vi "READ DUBAS DATA.vi"(7 "STATES":T1=enum."CLOSE", 8 "error in (no error)":errorcluster) -> (0 "error out":errorcluster, 3 "BUBAS DATA":dbl[](array[numeric]) caption="data" format="%.2f")   [LabVIEW 2018]
uses:
  Controls/DUBAS FGV STATES.ctl
  <vilib>/xnet/xnet.llb/XNET Create Session (Signal Input Single-point).vi
  <vilib>/xnet/xnet.llb/XNET Read (Signal Single-point).vi
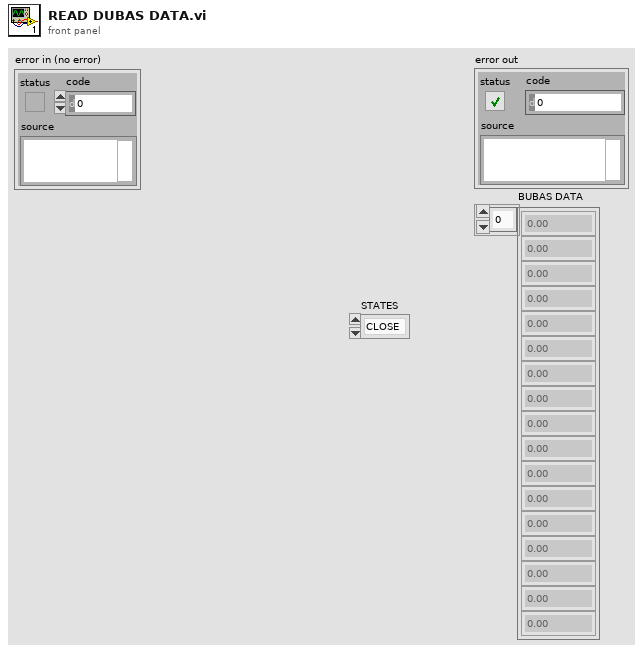
[diagram p1: front panel]
types:
  T1 = typedef "DUBAS FGV STATES.ctl" = enum16{"OPEN REF", "READ DATA", "CLOSE"}
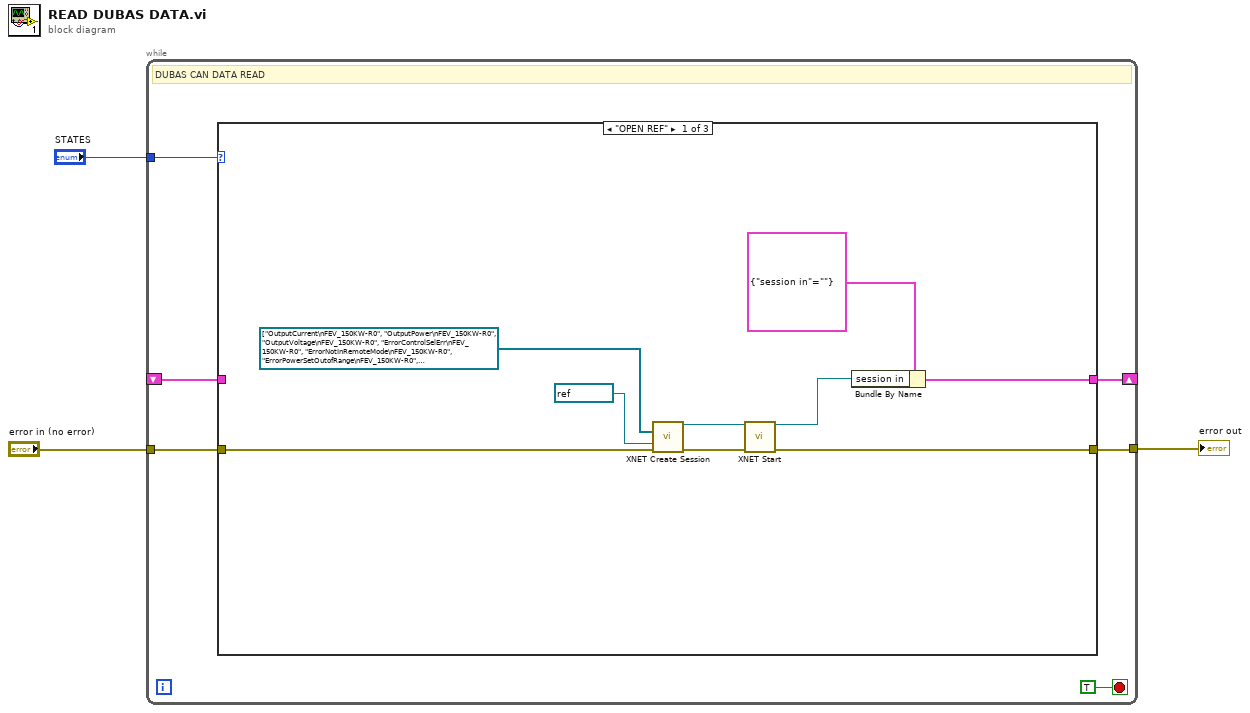
[diagram p0: block diagram]
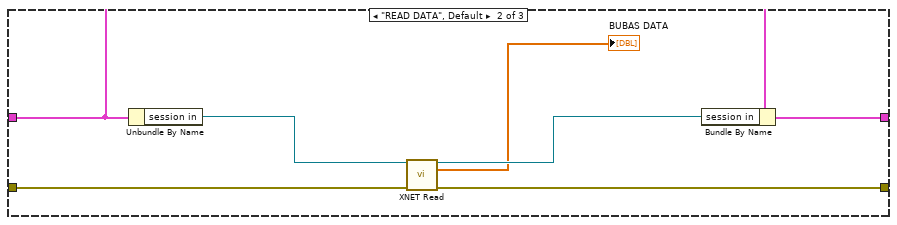
[diagram p2: hidden frame]
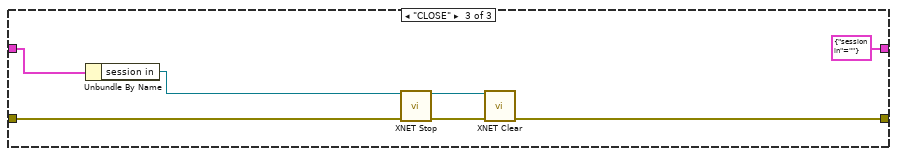
[diagram p3: hidden frame]
diagram:
  n1 = while {
    tunnel: "STATES" -> [w8]
    tunnel: "error in (no error)" -> [w7]
    tunnel: [w6] -> w1
    shift-right: [w5] -> _
    shift-left: _ -> [w4]
    stop <- TRUE stop-if-true
    # "DUBAS CAN DATA READ"
    n2 = case shown="\"OPEN REF\"" w8 {
      tunnel: w7 -> [w14 w25 w32]
      tunnel: [w13 w24 w27] -> w6
      tunnel: [w10 w20 cluster{"session in":refnum<k21>} {"session in"=""}] -> w5
      tunnel: w4 -> [_ w22 w31]
      frame "OPEN REF" {
        n3 = call-poly <vilib>:"XNET Create Session.vi"("signal list"=refnum<k21>[] ["OutputCurrent\nFEV_150KW-R0", "OutputPower\nFEV_150KW-R0", "OutputVoltage\nFEV_150KW-R0", "ErrorControlSelErr\nFEV_150KW-R0", "ErrorNotInRemoteMode\nFEV_150KW-R0", "ErrorPowerSetOutofRange\nFEV_150KW-R0", "ErrorVoltSetOutofRange\nFEV_150KW-R0", "ErrorWrongHVSel\nFEV_150KW-R0", "PowerSwitchONStatus\nFEV_150KW-R0", "StatusDcpsFault\nFEV_150KW-R0", "StatusHCHV_selection\nFEV_150KW-R0", "HandShakeAcknowledge\nFEV_150KW-R0", "RemoteDisplaySelAck\nFEV_150KW-R0", "Select_CVCICPAck\nFEV_150KW-R0", "Select_HVHC_Ack\nFEV_150KW-R0", "CV_SetCurrentLimitAck\nFEV_150KW-R0", "CV_SetPowerLimitAck\nFEV_150KW-R0", "CV_SetVoltageAck\nFEV_150KW-R0", "UpdateCmdAcknowledge\nFEV_150KW-R0"] ("Sigs 2"), "interface"=refnum<k21> "CAN2" ("Select Interface"), "error in (no error)"=w14) -> ("session out"=w17:refnum<k21>, "error out"=w18:errorcluster)  [unwired: 1 in, 10 out]
        n4 = call <vilib>:"XNET Start.vi"("session in"=w17, "error in (no error)"=w18) -> ("session out"=w11:refnum<k21>, "error out"=w13:errorcluster)  [unwired: 12 in]
        n5 = Bundle By Name(cluster=cluster{"session in":refnum<k21>} {"session in"=""}, "session in"=w11) -> (w10:cluster{"session in":refnum<k21>})
      }
      frame "READ DATA", Default {
        n6 = Unbundle By Name(w22) -> ("session in"=w23:refnum<k21>)
        n7 = call-poly <vilib>:"XNET Read.vi"("session in"=w23, "error in (no error)"=w25) -> ("session out"=w21:refnum<k21>, "data"=→"BUBAS DATA":dbl[], "error out"=w24:errorcluster)  [unwired: 11 in]
        n8 = Bundle By Name(cluster=w22, "session in"=w21) -> (w20:cluster{"session in":refnum<k21>})
      }
      frame "CLOSE" {
        n9 = Unbundle By Name(w31) -> ("session in"=w30:refnum<k21>)
        n10 = call <vilib>:"XNET Stop.vi"("session in"=w30, "error in (no error)"=w32) -> ("session out"=w29:refnum<k21>, "error out"=w28:errorcluster)  [unwired: 12 in]
        n11 = call <vilib>:"XNET Clear.vi"("session in"=w29, "error in (no error)"=w28) -> ("error out"=w27:errorcluster)  [unwired: 13 in]
      }
    }
  }
  "error out" <- w1
